vi "practica3tf.vi"() -> ()   [LabVIEW 2016]
panel:
  out "derecho Chart 2":dbl[](graph)
  out "izquierdo Chart":dbl[](graph)
  in  "stop":bool
  out "md":dbl(knob) scale=-100.0..100.0
  out "mi":dbl(knob) scale=-100.0..100.0
  in  "distancia":dbl(slide) scale=0.0..100.0
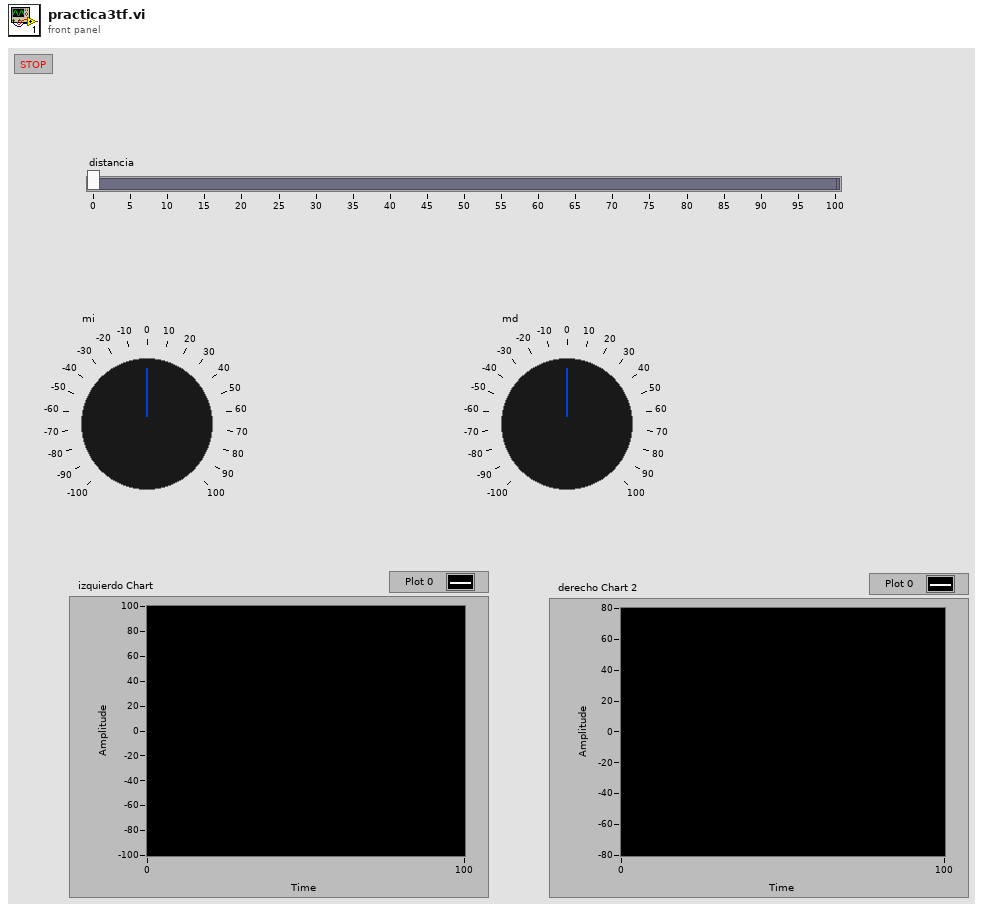
[diagram p1: front panel]
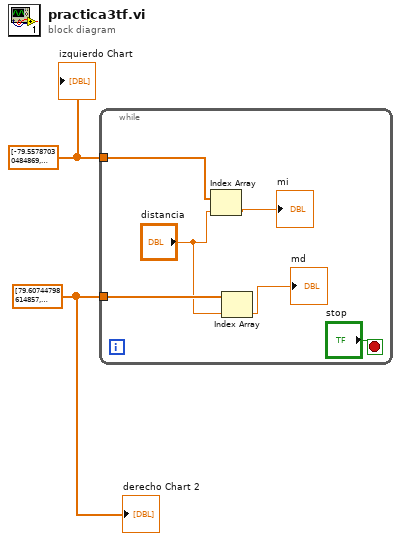
[diagram p0: block diagram]
diagram:
  w1 = dbl[] [79.60744798614857, 79.60744798614857, 79.60744798614857, 79.60744798614857, 79.60744798614857, 79.60744798614857, 79.60744798614857, 79.60744798614857, 79.60744798614857, 79.60744798614857, 79.60744798614857, 73.9327945943478, 67.74600746758951, 59.948267960006014, 49.03069934659603, 35.04240405839756, 34.997269472704836, 35.00417610132282, 35.003676510936245, 35.011068647642546, 35.01222409099579, 34.99804181827941, 35.011282295932794, 35.004585293041345, 35.00611464305229, 35.003315405584615, 35.00611464305229, 35.004585293041345, 35.011282295932794, 34.99804181827941, 35.01222409099579, 35.011068647642546, 35.003676510936245, 35.00417610132282, 34.997269472704836, 35.04240405839756, 34.968998996537735, 35.048132460531384, 35.048132460531384, 34.968998996537735, 35.04240405839756, 34.997269472704836, 35.00417610132282, 35.003676510936245, 35.011068647642546, 35.01222409099579, 34.99804181827941, 35.011282295932794, 35.004585293041345, 35.00611464305229, 35.003315405584615, 29.957381592629172, 25.549601933486095, 21.75934839548812, 18.12306491123468, 14.70968278950392, 11.603545456917844, 8.45898270355057, 4.993514411221481, 1.4506880794304629, -2.437901491227444, -6.830683096134281, -11.815837039055035, -17.85404342499758, -25.03720771651005, -34.97143473936609, -34.96057345546029, -34.9902236651717, -34.983218240037026, -34.97791759461981, -34.983218240037026, -34.97860289072147, -34.977809408870485, -34.98412301495825, -34.98321824003704, -34.98251521823598, -34.98382079524988, -34.97560693116882, -34.983218240037026, -34.98095612449242, -34.99263480383682, -34.97143473936609, -34.97740310774286, -34.98866739904417, -34.935632693353746, -34.97402774265092, -49.06373285357404, -59.86617522234936, -67.68957691254778, -73.99944426373509, -79.55787030484869, -79.55787030484869, -79.55787030484869, -79.55787030484869, -79.55787030484869, -79.55787030484869, -79.55787030484869, -79.55787030484869, -79.55787030484869, -79.55787030484869] ("Waveform Chart 2")
  w2 = dbl[] [-79.55787030484869, -79.55787030484869, -79.55787030484869, -79.55787030484869, -79.55787030484869, -79.55787030484869, -79.55787030484869, -79.55787030484869, -79.55787030484869, -79.55787030484869, -79.55787030484869, -73.99944426373509, -67.68957691254778, -59.86617522234936, -49.06373285357404, -34.97402774265092, -34.935632693353746, -34.98866739904417, -34.97740310774286, -34.97143473936609, -34.99263480383682, -34.98095612449242, -34.983218240037026, -34.97560693116882, -34.98382079524988, -34.98251521823598, -34.98382079524988, -34.97560693116882, -34.983218240037026, -34.98095612449242, -34.99263480383682, -34.97143473936609, -34.97740310774286, -34.98866739904417, -34.935632693353746, -34.97402774265092, -19.261843421646017, -6.522316530395521, 6.4889232641317935, 19.78710856443898, 35.04240405839756, 34.997269472704836, 35.00417610132282, 35.003676510936245, 35.011068647642546, 35.01222409099579, 34.99804181827941, 35.011282295932794, 35.004585293041345, 35.00611464305229, 35.003315405584615, 35.00611464305229, 35.004585293041345, 35.011282295932794, 34.99804181827941, 35.01222409099579, 35.011068647642546, 35.003676510936245, 35.00417610132282, 34.997269472704836, 34.997269472704836, 35.017294733851905, 34.99800794591345, 34.980892012244034, 35.02326283573281, 35.011068647642546, 34.999745110367215, 35.00928280967127, 35.00077627323856, 34.995471018032305, 35.011282295932794, 35.007229893129754, 35.00513637083321, 35.0067662174107, 35.004819601786885, 35.003315405584615, 35.00611464305229, 35.004585293041345, 35.011282295932794, 34.99804181827941, 35.01222409099579, 35.011068647642546, 35.003676510936245, 35.00417610132282, 34.997269472704836, 35.04240405839756, 49.03069934659603, 59.948267960006014, 67.74600746758951, 73.9327945943478, 79.60744798614857, 79.60744798614857, 79.60744798614857, 79.60744798614857, 79.60744798614857, 79.60744798614857, 79.60744798614857, 79.60744798614857, 79.60744798614857, 79.60744798614857] ("Waveform Chart")
  n1 = while {
    tunnel: w2 -> [w8]
    tunnel: w1 -> [w7]
    stop <- "stop" stop-if-true
    n2 = Index Array(array=w8, index="distancia") -> (element=→"mi":dbl)
    n3 = Index Array(array=w7, index="distancia") -> (element=→"md":dbl)
  }
  "izquierdo Chart" <- w2
  "derecho Chart 2" <- w1
